vi "test1.vi"() -> ()   [LabVIEW 2020]
uses:
  <vilib>/Instr/_visa.llb/VISA Configure Serial Port (Instr).vi
panel:
  in  "Boolean":bool
  out "XY Graph":cluster{"X":dbl, "Y":dbl}[](graph)
  out "Angle":dbl(knob) scale=-25.0..25.0
  in  "START":bool
  out "Waveform Chart":dbl(graph)
  out "read buffer":string
  in  "VISA resource name":refnum<visa-resource-name>
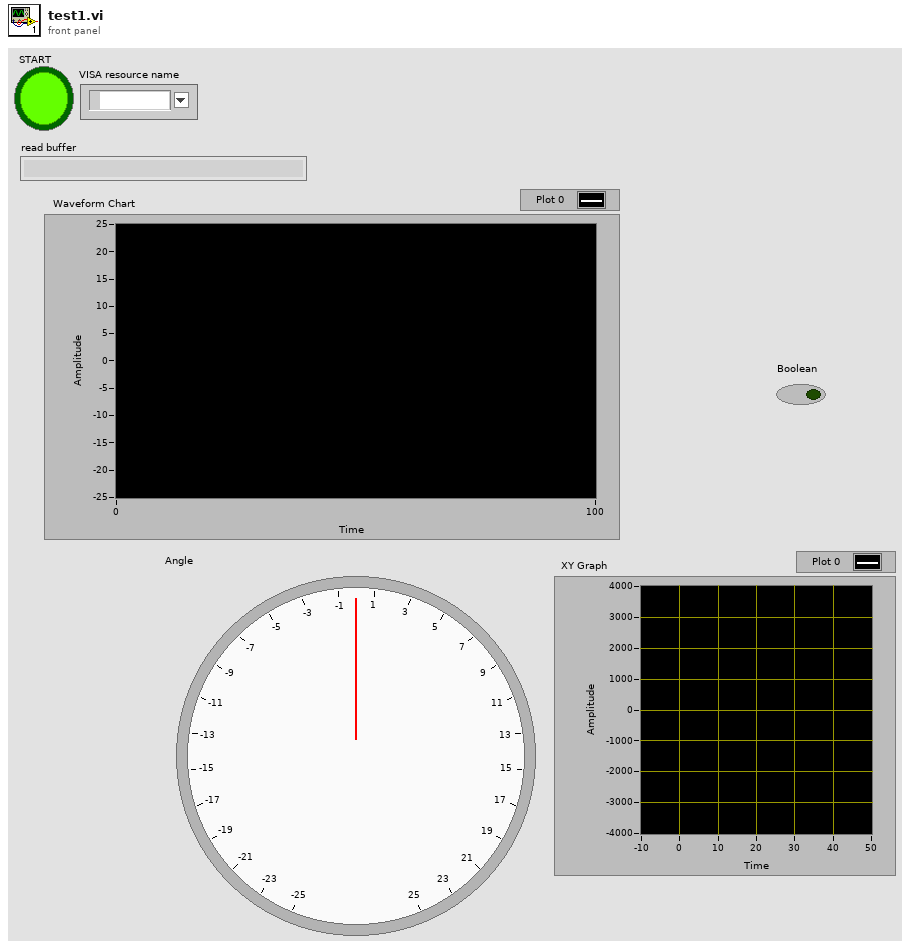
[diagram p1: front panel]
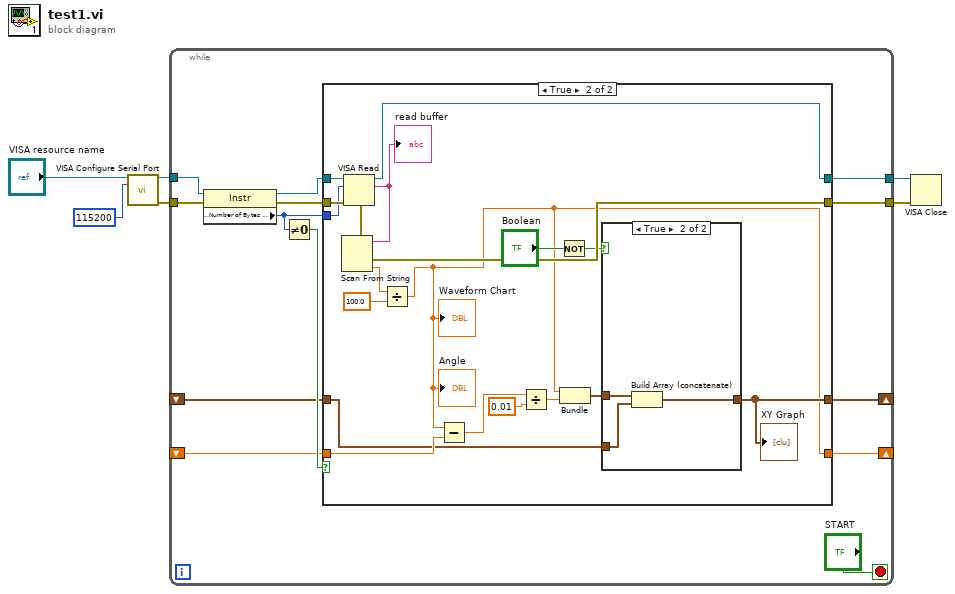
[diagram p0: block diagram]
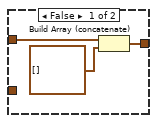
[diagram p3: hidden frame]
diagram:
  n1 = call-poly "VISA Configure Serial Port"("VISA resource name"="VISA resource name", "baud rate (9600)"=u32 115200) -> ("VISA resource name out"=w5:refnum<visa-resource-name>, "error out"=w4:errorcluster)  [unwired: 12 in]
  n2 = while {
    tunnel: w5 -> [w18]
    tunnel: w4 -> [w19]
    tunnel: [w15] -> w2
    tunnel: [w14] -> w1
    shift-right: [w10] -> _
    shift-left: _ -> [w9]
    shift-right: [w8] -> _
    shift-left: _ -> [w7]
    stop <- "START" stop-if-true
    n3 = property class="Instr"(reference=w18, error in=w19) -> (reference out=w16:refnum<visa-resource-name>, error out=w17:errorcluster, "Serial Settings:Number of Bytes at Serial Port"=w12:u32)
    n4 = Not Equal To 0?(x=w12) -> (x != 0?=w13:bool)
    n5 = case shown="True" w13 {
      tunnel: w17 -> [w22 w42]
      tunnel: w16 -> [w23 w41]
      tunnel: w12 -> [_ w40]
      tunnel: [w23 w37] -> w15
      tunnel: [w22 w36] -> w14
      tunnel: [w21 w25] -> w10
      tunnel: w9 -> [w21 w35]
      tunnel: [w20 w29] -> w8
      tunnel: w7 -> [w20 w30]
      frame False {
      }
      frame True {
        n6 = VISA Read(VISA resource name=w41, byte count=w40, error in (no error)=w42) -> (VISA resource name out=w37:refnum<visa-resource-name>, read buffer=w39:string, error out=w38:errorcluster)  [unwired: 1 out]
        "read buffer" <- w39
        n7 = Scan From String(input string=w39, error in=w38) -> (error out=w36:errorcluster, output 1=w26:dbl)  [unwired: 3 in, 2 out]
        n8 = Divide(x=w26, y=100.0) -> (x/y=w25:dbl)
        "Waveform Chart" <- w25
        "Angle" <- w25
        n9 = Subtract(x=w25, y=w35) -> (x-y=w34:dbl)
        n10 = Divide(x=w34, y=0.01) -> (x/y=w32:dbl)
        n11 = Not(x="Boolean") -> (.not. x?=w27:bool)
        n12 = Bundle(w25, w32) -> (w31:cluster{dbl, dbl})  [unwired: 1 in]
        n13 = case shown="True" w27 {
          tunnel: w31 -> [w45 w48]
          tunnel: w30 -> [_ w47]
          tunnel: [w43 w46] -> w29
          frame False {
            n14 = Build Array (concatenate)(w45, cluster{"Waveform Chart":dbl, dbl}[] [] ("array")) -> (w43:cluster{"Waveform Chart":dbl, dbl}[])
          }
          frame True {
            n15 = Build Array (concatenate)(w48, w47) -> (w46:cluster{"Waveform Chart":dbl, dbl}[])
          }
        }
        "XY Graph" <- w29
      }
    }
  }
  n16 = VISA Close(VISA resource name=w2, error in (no error)=w1) -> ()  [unwired: 1 out]
